vi "PID-rodolfo-1c.vi"(4 "output range":cluster{"output high":i16, "output low":i16}={"output high"=32767, "output low"=-32768}, 5 "shift integrator":i32, 7 "P scale":i8=-1, 8 "PID gains (x 2^8)":T1={"proportional gain (Kc)"=1, "integral gain (Kc*Ts/Ti)"=0, "derivative gain (Kc*Td/Ts)"=0}, 9 "I scale":i8, 10 "process variable":i16, 11 "setpoint":i16) -> (0 "yes/no":bool, 1 "upper/lower":bool, 2 "output":i16)   [LabVIEW 2012]
uses:
  <vilib>/rvi/Arithmetic/AddSubMult/XNode/nirviSatArithmetic.xnode
panel:
  in  "initialize":bool
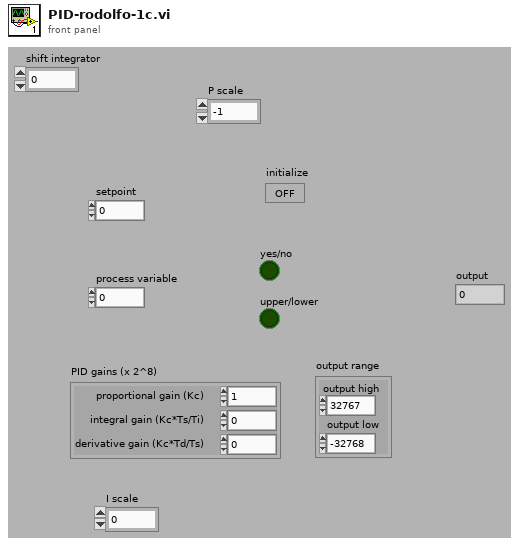
[diagram p1: front panel]
types:
  T1 = cluster{"proportional gain (Kc)":i16, "integral gain (Kc*Ts/Ti)":i16, "derivative gain (Kc*Td/Ts)":i16}
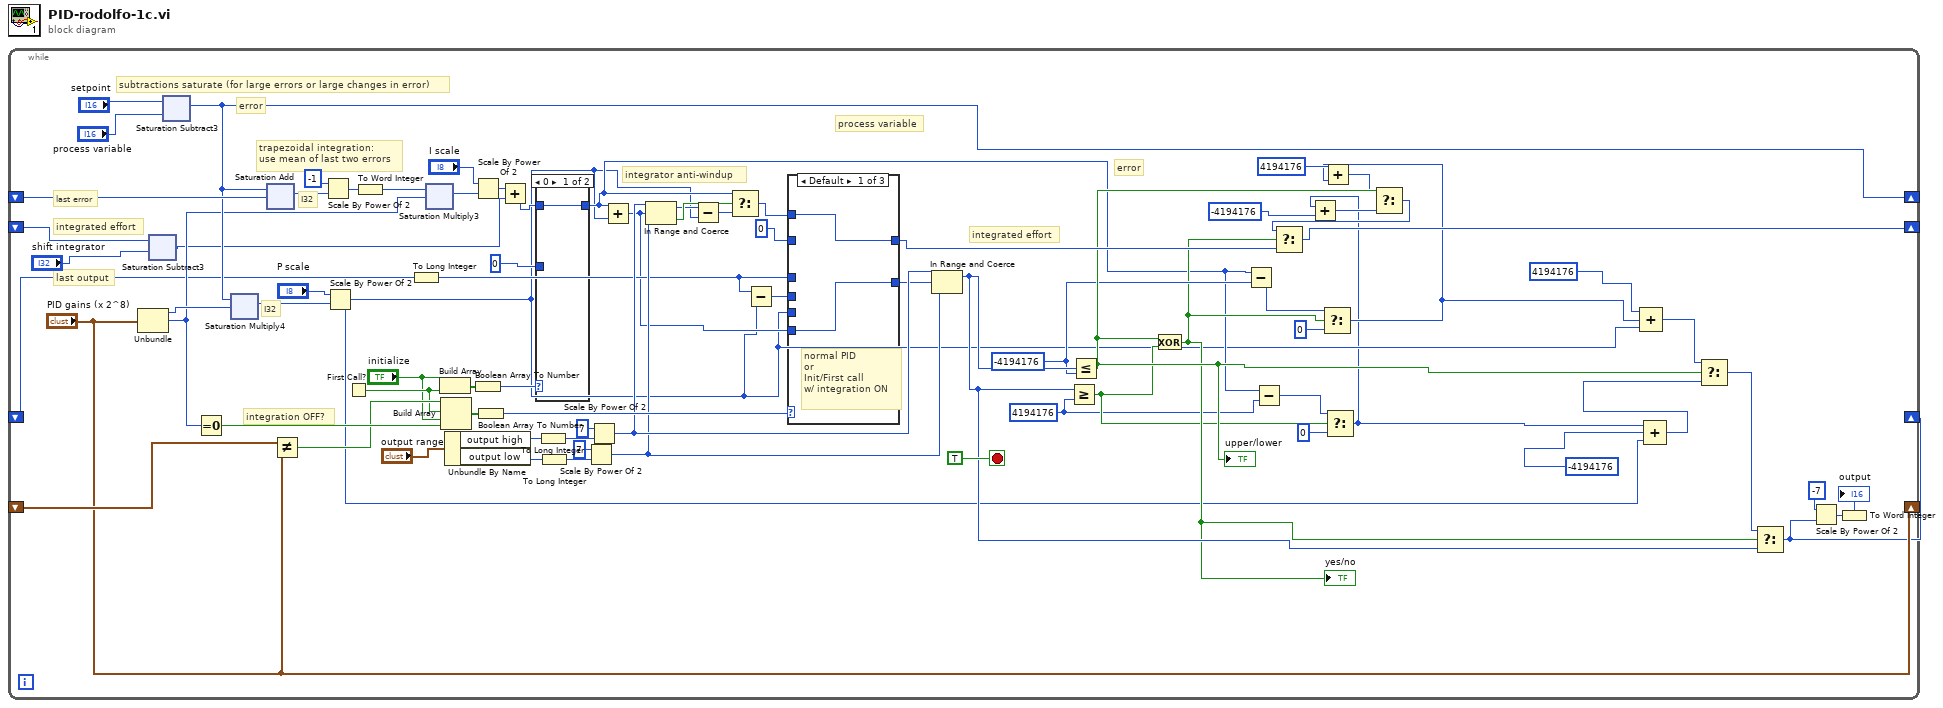
[diagram p0: block diagram]
diagram:
  n1 = while {
    shift-right: [w35] -> _
    shift-left: _ -> [w33]
    shift-right: [w50] -> _
    shift-left: _ -> [w58]
    shift-right: [w34] -> _
    shift-left: _ -> [w3]
    shift-right: ["PID gains (x 2^8)"] -> _
    shift-left: _ -> [w79]
    stop <- TRUE stop-if-true
    w17 = -4194176 ("y")
    w9 = 4194176 ("y")
    # "I32"
    # "I32"
    # "integration OFF?"
    # "integrator anti-windup"
    # "last output"
    # "integrated effort"
    # "trapezoidal integration:\nuse mean of last two errors"
    # "error"
    # "subtractions saturate (for large errors or large changes in error)"
    # "last error"
    # "error"
    # "process variable"
    # "integrated effort"
    n2 = Unbundle("PID gains (x 2^8)") -> ("proportional gain (Kc)"=w54:i16, "integral gain (Kc*Ts/Ti)"=w36:i16)  [unwired: 1 out]
    n3 = xnode ("Saturation Subtract3")("x"=w3, "y"="shift integrator") -> ("x-y"=w1:i32)
    n4 = xnode ("Saturation Subtract3")("x"="setpoint", "y"="process variable") -> ("x-y"=w50:i16)
    n5 = Equal To 0?(x=w36) -> (x = 0?=w73:bool)
    n6 = xnode ("Saturation Multiply4")("x"=w50, "y"=w54) -> ("x*y"=w53:i32)
    n7 = xnode ("Saturation Add")("x"=w50, "y"=w58) -> ("x+y"=w57:i32)
    n8 = Not Equal?(x=w79, y="PID gains (x 2^8)") -> (x != y?=w39:bool)
    n9 = Scale By Power Of 2(n=i8 -1, x=w57) -> (x*2^n=w76:i32)
    n10 = Scale By Power Of 2(n="P scale", x=w53) -> (x*2^n=w5:i32)
    n11 = First Call?() -> (First Call?: T/F=w38:bool)
    n12 = To Word Integer(number=w76) -> (16bit integer=w56:i16)
    n13 = To Long Integer(number=w33) -> (32bit integer=w31:i32)
    n14 = xnode ("Saturation Multiply3")("x"=w56, "y"=w36) -> ("x*y"=w55:i32)
    n15 = Build Array("initialize", w38) -> (w62:bool[])
    n16 = Build Array(w39, w38, "initialize", w73) -> (w72:bool[])
    n17 = Unbundle By Name("output range") -> ("output high"=w65:i16, "output low"=w45:i16)
    n18 = Scale By Power Of 2(n="I scale", x=w55) -> (x*2^n=w74:i32)
    n19 = Boolean Array To Number(Boolean array=w62) -> (number=w61:u8)
    n20 = Boolean Array To Number(Boolean array=w72) -> (number=w71:u8)
    n21 = Add(x=w74, y=w1) -> (x+y=w60:i32)
    n22 = case shown="0" w61 {
      tunnel: w60 -> [w159 _]
      tunnel: [w159 w160] -> w8
      tunnel: 0 ("t") -> [_ w160]
      frame 0 {
      }
      frame Default {
        # "Init/\nFirst call"
      }
    }
    n23 = To Long Integer(number=w65) -> (32bit integer=w47:i32)
    n24 = To Long Integer(number=w45) -> (32bit integer=w44:i32)
    n25 = Scale By Power Of 2(n=7, x=w44) -> (x*2^n=w43:i32)
    n26 = Scale By Power Of 2(n=7, x=w47) -> (x*2^n=w49:i32)
    n27 = Add(x=w8, y=w5) -> (x+y=w29:i32)
    n28 = In Range and Coerce(upper limit=w49, x=w29, lower limit=w43) -> (coerced(x)=w66:i32, In Range?=w67:bool)
    n29 = Subtract(x=w66, y=w5) -> (x-y=w68:i32)
    n30 = Select(t=w8, s=w67, f=w68) -> (s? t:f=w64:i32)
    n31 = Subtract(x=w31, y=w5) -> (x-y=w70:i32)
    n32 = case shown="Default" w71 {
      tunnel: [w161 w164 w165] -> w32
      tunnel: [w162 w163 w166] -> w24
      tunnel: w5 -> [_ _ w166]
      tunnel: w70 -> [_ w164 _]
      tunnel: w29 -> [w162 _ _]
      tunnel: w64 -> [w161 _ _]
      tunnel: w31 -> [_ w163 _]
      tunnel: 0 ("t") -> [_ _ w165]
      frame Default {
        # "normal PID\nor\nInit/First call\nw/ integration ON"
      }
      frame 1 {
        # "last output - (P+D)"
        # "last output"
        # "PID gains have \nchanged since last iteration"
        # "P+D"
      }
      frame 8.. {
        # "0"
        # "P+D"
        # "Integration OFF"
      }
    }
    n33 = In Range and Coerce(upper limit=w49, x=w24, lower limit=w43) -> (coerced(x)=w25:i32)  [unwired: 1 out]
    n34 = Greater Or Equal?(x=w25, y=w9) -> (x >= y?=w10:bool)
    n35 = Less Or Equal?(x=w25, y=w17) -> (x <= y?=w27:bool)
    "upper/lower" <- w27
    n36 = Exclusive Or(1:w10, 2:w27) -> (0:w15:bool)
    "yes/no" <- w15
    n37 = Subtract(x=w8, y=w17) -> (x-y=w16:i32)
    n38 = Subtract(x=w8, y=w9) -> (x-y=w7:i32)
    n39 = Select(t=w16, s=w15, f=0) -> (s? t:f=w14:i32)
    n40 = Add(x=4194176, y=w14) -> (x+y=w20:i32)
    n41 = Select(t=w7, s=w10, f=0) -> (s? t:f=w4:i32)
    n42 = Add(x=w4, y=-4194176) -> (x+y=w18:i32)
    n43 = Select(t=w20, s=w27, f=w18) -> (s? t:f=w28:i32)
    n44 = Select(t=w28, s=w15, f=w32) -> (s? t:f=w34:i32)
    n45 = Compound Arithmetic op=ADD(4194176, w14, w5) -> (w22:i32)
    n46 = Compound Arithmetic op=ADD(w4, -4194176 ("t"), w5) -> (w11:i32)
    n47 = Select(t=w22, s=w27, f=w11) -> (s? t:f=w26:i32)
    n48 = Select(t=w26, s=w15, f=w25) -> (s? t:f=w35:i32)
    n49 = Scale By Power Of 2(n=-7, x=w35) -> (x*2^n=w41:i32)
    n50 = To Word Integer(number=w41) -> (16bit integer=→"output":i16)
  }
